vi "List Folder.vi"(8 "error in (no error)":errorcluster, 11 "path":path) -> (0 "error out":errorcluster)   [LabVIEW 2018, in "LogonUser.lvclass"]
doc: "©2019\nWiebe Walstra\nwww.carya.nl"
uses:
  LogonUser.lvclass
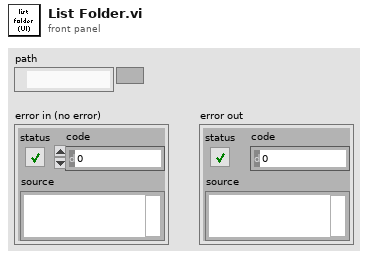
[diagram p1: front panel]
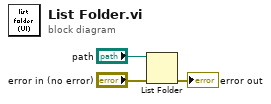
[diagram p0: block diagram]
diagram:
  n1 = List Folder(path="path", error in="error in (no error)") -> (error out=→"error out":errorcluster)  [unwired: 2 in, 3 out]
